vi "TestAll.vi"(8 "error in (no error)":errorcluster) -> (0 "error out":errorcluster, 3 "report":string)   [LabVIEW 2018]
uses:
  <vilib>/addons/_JKI Toolkits/Caraya/classes/Test Suite/Define Test Suite (SimpleText Report).vi
  <vilib>/addons/_JKI Toolkits/Caraya/classes/Test Suite/Test Suite.lvclass
panel:
  out "Succeeded?":bool
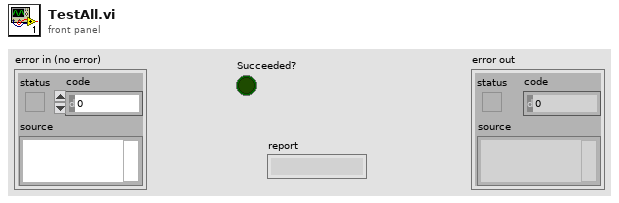
[diagram p1: front panel]
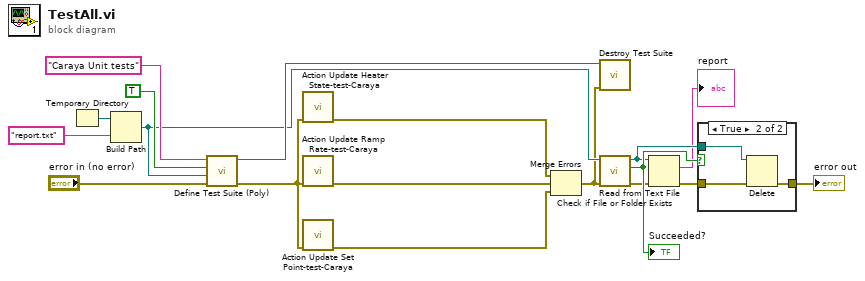
[diagram p0: block diagram]
diagram:
  n1 = Temporary Directory() -> (w14:path)
  n2 = Build Path(base path=w14, name or relative path="report.txt") -> (appended path=w8:path)
  n3 = call-poly <vilib>:"Define Test Suite (Poly).vi"("error in (no error)"="error in (no error)", "Report Path"=w8, "Interactive"=TRUE, "Label (VI Title)"="Caraya Unit tests") -> ("error out"=w1:errorcluster, "Test Suite"=w16:refnum<class "Test Suite.lvclass">)  [unwired: 6 in]
  n4 = call "Action Update Heater State-test-Caraya.vi"("error in (no error)"=w1) -> ("error out"=w4:errorcluster)  [unwired: 10 in]
  n5 = call "Action Update Ramp Rate-test-Caraya.vi"("error in (no error)"=w1) -> ("error out"=w3:errorcluster)  [unwired: 10 in]
  n6 = call "Action Update Set Point-test-Caraya.vi"("error in (no error)"=w1) -> ("error out"=w2:errorcluster)  [unwired: 10 in]
  n7 = Merge Errors(w4, w3, w2) -> (w7:errorcluster)
  n8 = call-dynamic "Destroy Test Suite.vi"("error in (no error)"=w7, "Test Suite in"=w16) -> ()  [unwired: 9 in, 1 out]
  n9 = call <vilib>:"Check if File or Folder Exists.vi"("error in (no error)"=w7, "path"=w8) -> ("error out"=w11:errorcluster, "file or folder exists?"=w12:bool, "dup path"=w9:path)  [unwired: 7 in]
  "Succeeded?" <- w12
  n10 = Read from Text File(file (use dialog)=w9, error in=w11) -> (text=→"report":string, error out=w10:errorcluster)  [unwired: 2 in, 2 out]
  n11 = case shown="True" w12 {
    tunnel: w9 -> [_ w22]
    tunnel: w10 -> [w19 w21]
    tunnel: [w19 w20] -> w6
    frame False {
    }
    frame True {
      n12 = Delete(path (use dialog)=w22, error in=w21) -> (error out=w20:errorcluster)  [unwired: 3 in, 2 out]
    }
  }
  "error out" <- w6
